vi "AddIndicatorToReadVI.vi"(8 "error in (no error)":errorcluster, 11 "BaseAccessorScripter in":refnum<class "BaseAccessorScripter.lvclass">) -> (0 "error out":errorcluster, 3 "BaseAccessorScripter out":refnum<class "BaseAccessorScripter.lvclass">)   [LabVIEW 2021, in "MemberVICreation.lvlib" / "BaseAccessorScripter.lvclass"]
uses:
  <resource>/Framework/Providers/LVClassLibrary/NewAccessors/BaseAccessorScripter/BaseAccessorScripter.lvclass
  <resource>/Framework/Providers/LVClassLibrary/NewAccessors/BaseAccessorScripter/BaseAccessorScripter.lvclass/BaseAccessorScripter.ctl
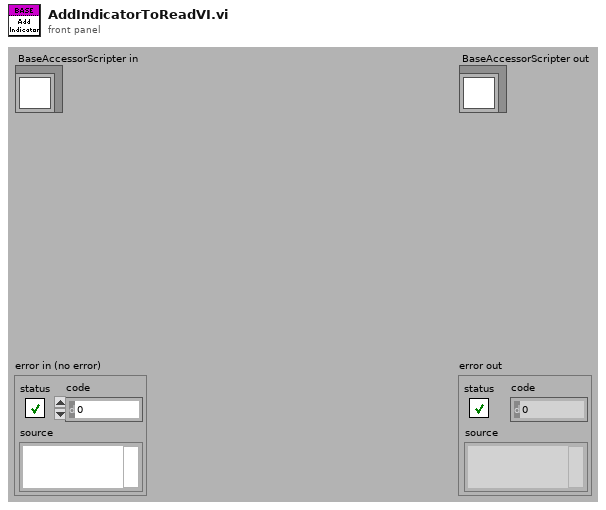
[diagram p1: front panel]
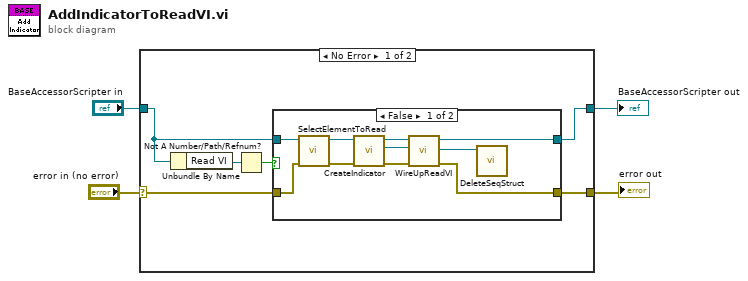
[diagram p0: block diagram]
diagram:
  n1 = case shown="No Error" "error in (no error)" {
    selector: "error in (no error)" -> [w7 w24]
    tunnel: [w5 w24] -> w3
    tunnel: [w6 w23] -> w1
    tunnel: "BaseAccessorScripter in" -> [w8 w23]
    frame No Error {
      n2 = Unbundle By Name(w8) -> ("Read VI"=w10:refnum<vi>)
      n3 = Not A Number/Path/Refnum?(number/path/refnum=w10) -> (NaN/Path/Refnum?=w9:bool)
      n4 = case shown="False" w9 {
        tunnel: w8 -> [w16 w22]
        tunnel: w7 -> [w15 w21]
        tunnel: [w19 w22] -> w6
        tunnel: [w11 w21] -> w5
        frame False {
          n5 = call-dynamic "SelectElementToRead.vi"("error in (no error)"=w15, "BaseAccessorScripter in"=w16) -> ("error out"=w14:errorcluster, "BaseAccessorScripter out"=w13:refnum<class "BaseAccessorScripter.lvclass">)  [unwired: 8 out]
          n6 = call-dynamic "CreateIndicator.vi"("error in (no error)"=w14, "BaseAccessorScripter in"=w13) -> ("error out"=w18:errorcluster, "New Control Ref"=w17:refnum<vi>, "BaseAccessorScripter out"=w20:refnum<class "BaseAccessorScripter.lvclass">)  [unwired: 7 out]
          n7 = call-dynamic "WireUpReadVI.vi"("error in (no error)"=w18, "New Control Ref"=w17, "BaseAccessorScripter in"=w20) -> ("error out"=w11:errorcluster, "Multiframe Stuct out"=w12:refnum<vi>, "BaseAccessorScripter out"=w19:refnum<class "BaseAccessorScripter.lvclass">)  [unwired: 6 out]
          n8 = call <resource>:"DeleteSeqStruct.vi"("Multiframe Stuct in"=w12) -> ()  [unwired: 1 in, 8 out]
        }
        frame True {
        }
      }
    }
    frame Error {
    }
  }
  "error out" <- w3
  "BaseAccessorScripter out" <- w1
